vi "RichToFlatnixnet_grpc_CreateSessionRequest.vi"(5 "OutputClusterType":T1, 11 "InputCluster":T4) -> (3 "OutputCluster":T1)   [LabVIEW 2024, in "grpc-xnet_client.lvlib"]
uses:
  grpc-xnet_client.lvlib
  nixnet_grpc_CreateSessionRequest_mode_enum/nixnet_grpc_CreateSessionRequest_mode_enum.lvclass
  nixnet_grpc_CreateSessionRequest_mode_enum/nixnet_grpc_CreateSessionRequest_mode_enum.lvclass/nixnet_grpc_CreateSessionRequest_mode_enum.ctl
  nidevice_grpc_SessionInitializationBehavior.ctl
  nixnet_grpc_CreateSessionMode.ctl
  nixnet_grpc_CreateSessionRequest_Flat.ctl
  nixnet_grpc_CreateSessionRequest.ctl
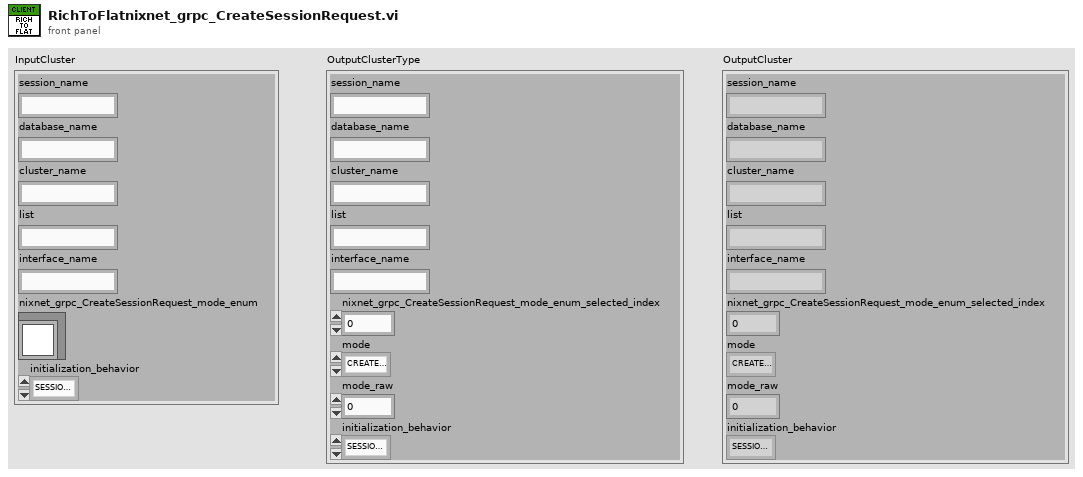
[diagram p1: front panel]
types:
  T1 = typedef "grpc-xnet_client.lvlib/nixnet_grpc_CreateSessionRequest_Flat.ctl" = cluster{"session_name":string, "database_name":string, "cluster_name":string, "list":string, "interface_name":string, "nixnet_grpc_CreateSessionRequest_mode_enum_selected_index":i32, "mode":T2, "mode_raw":u32, "initialization_behavior":T3}
  T2 = typedef "grpc-xnet_client.lvlib/nixnet_grpc_CreateSessionMode.ctl" = enum32{"CREATE_SESSION_MODE_SIGNAL_IN_SINGLE_POINT", "CREATE_SESSION_MODE_SIGNAL_IN_WAVEFORM", "CREATE_SESSION_MODE_SIGNAL_IN_XY", "CREATE_SESSION_MODE_SIGNAL_OUT_SINGLE_POINT", "CREATE_SESSION_MODE_SIGNAL_OUT_WAVEFORM", "CREATE_SESSION_MODE_SIGNAL_OUT_XY", "CREATE_SESSION_MODE_FRAME_IN_STREAM", "CREATE_SESSION_MODE_FRAME_IN_QUEUED", "CREATE_SESSION_MODE_FRAME_IN_SINGLE_POINT", "CREATE_SESSION_MODE_FRAME_OUT_STREAM", "CREATE_SESSION_MODE_FRAME_OUT_QUEUED", "CREATE_SESSION_MODE_FRAME_OUT_SINGLE_POINT", "CREATE_SESSION_MODE_SIGNAL_CONVERSION_SINGLE_POINT"}
  T3 = typedef "grpc-xnet_client.lvlib/nidevice_grpc_SessionInitializationBehavior.ctl" = enum32{"SESSION_INITIALIZATION_BEHAVIOR_UNSPECIFIED", "SESSION_INITIALIZATION_BEHAVIOR_INITIALIZE_NEW", "SESSION_INITIALIZATION_BEHAVIOR_ATTACH_TO_EXISTING"}
  T4 = typedef "grpc-xnet_client.lvlib/nixnet_grpc_CreateSessionRequest.ctl" = cluster{"session_name":string, "database_name":string, "cluster_name":string, "list":string, "interface_name":string, "nixnet_grpc_CreateSessionRequest_mode_enum":refnum<class "nixnet_grpc_CreateSessionRequest_mode_enum.lvclass">, "initialization_behavior":T3}
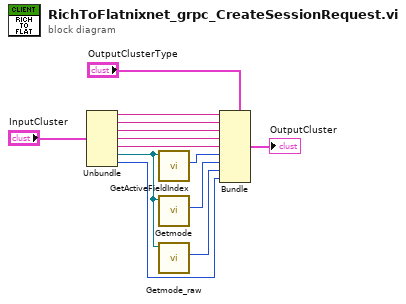
[diagram p0: block diagram]
diagram:
  n1 = Unbundle "Unbundle"("InputCluster") -> ("session_name"=w10:string, "database_name"=w9:string, "cluster_name"=w8:string, "list"=w7:string, "interface_name"=w6:string, "nixnet_grpc_CreateSessionRequest_mode_enum"=w5:refnum<class "nixnet_grpc_CreateSessionRequest_mode_enum.lvclass">, "initialization_behavior"=w1:T3)
  n2 = call "GetActiveFieldIndex.vi"("OneOfTemplate in"=w5) -> ("Active Field Index"=w4:i32)  [unwired: 8 in, 2 out]
  n3 = call "Getmode.vi"("OneOfTemplate in"=w5) -> ("Get_Val"=w3:T2)  [unwired: 8 in, 2 out]
  n4 = call "Getmode_raw.vi"("OneOfTemplate in"=w5) -> ("Get_Val"=w2:u32)  [unwired: 8 in, 2 out]
  n5 = Bundle "Bundle"(cluster="OutputClusterType", "session_name"=w10, "database_name"=w9, "cluster_name"=w8, "list"=w7, "interface_name"=w6, "nixnet_grpc_CreateSessionRequest_mode_enum_selected_index"=w4, "mode"=w3, "mode_raw"=w2, "initialization_behavior"=w1) -> (→"OutputCluster":T1)
